vi "CG_Auswertung.vi"() -> ()   [LabVIEW 2020, in "Erweiterte Konfig.lvlib" / "CG-Check Konfig.lvlib"]
uses:
  CG-Check Konfig.lvlib
  CalEingaenge.ctl
  System Einstellungen V2/Aktioen FGV System Konstanten.ctl
  Aktion_CG-Check.ctl
  <vilib>/Utility/miscctls.llb/LVRowAndColumnTypeDef.ctl
  FT-IR/Span/Spanfaktor.lvlib
  Allgemein/allgemeine Sub-VIs.lvlib
  Sprachverwaltung/Sprachverwaltung.lvlib
  System Einstellungen V2/System Einstellungen V2.lvlib
panel:
  in  "Abbrechen":bool
  in  "Register":T1(tab)
  in  "Tabelle Span 1":string[][](table)
  in  "Tabelle Span 2":string[][](table)
  in  "Tabelle Span 3":string[][](table)
  in  "Tabelle Cal Gas O2":string[][](table)
  # "CG-Test Ergebnis"
  # "Komponente"
  # "Komponente"
  # "Komponente"
  # "Komponente"
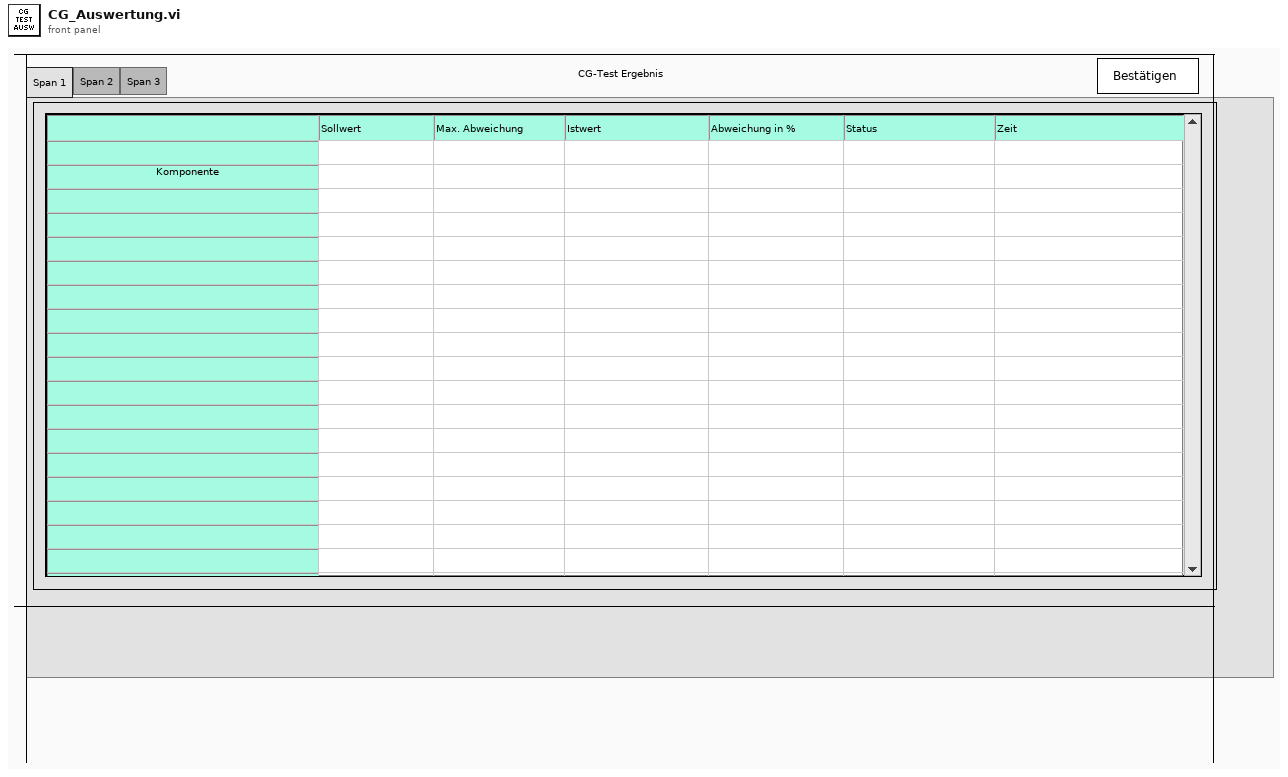
[diagram p1: front panel]
types:
  T1 = enum32{"Span 1", "Span 2", "Span 3", "Cal Gas O2"}
  T2 = typedef "System Einstellungen V2.lvlib/Aktioen FGV System Konstanten.ctl" = enum16{"lesen", "laden", "speichern", "Sprache"}
  T3 = typedef "Erweiterte Konfig.lvlib/CG-Check Konfig.lvlib/Aktion_CG-Check.ctl" = enum16{"lesen", "schreiben", "laden", "Komponente", "Aktive?", "speichern"}
  T4 = typedef "LVRowAndColumnTypeDef.ctl" = cluster{"Row":i32, "Column":i32}
  T5 = typedef "Erweiterte Konfig.lvlib/CG-Check Konfig.lvlib/CalEingaenge.ctl" = string[]
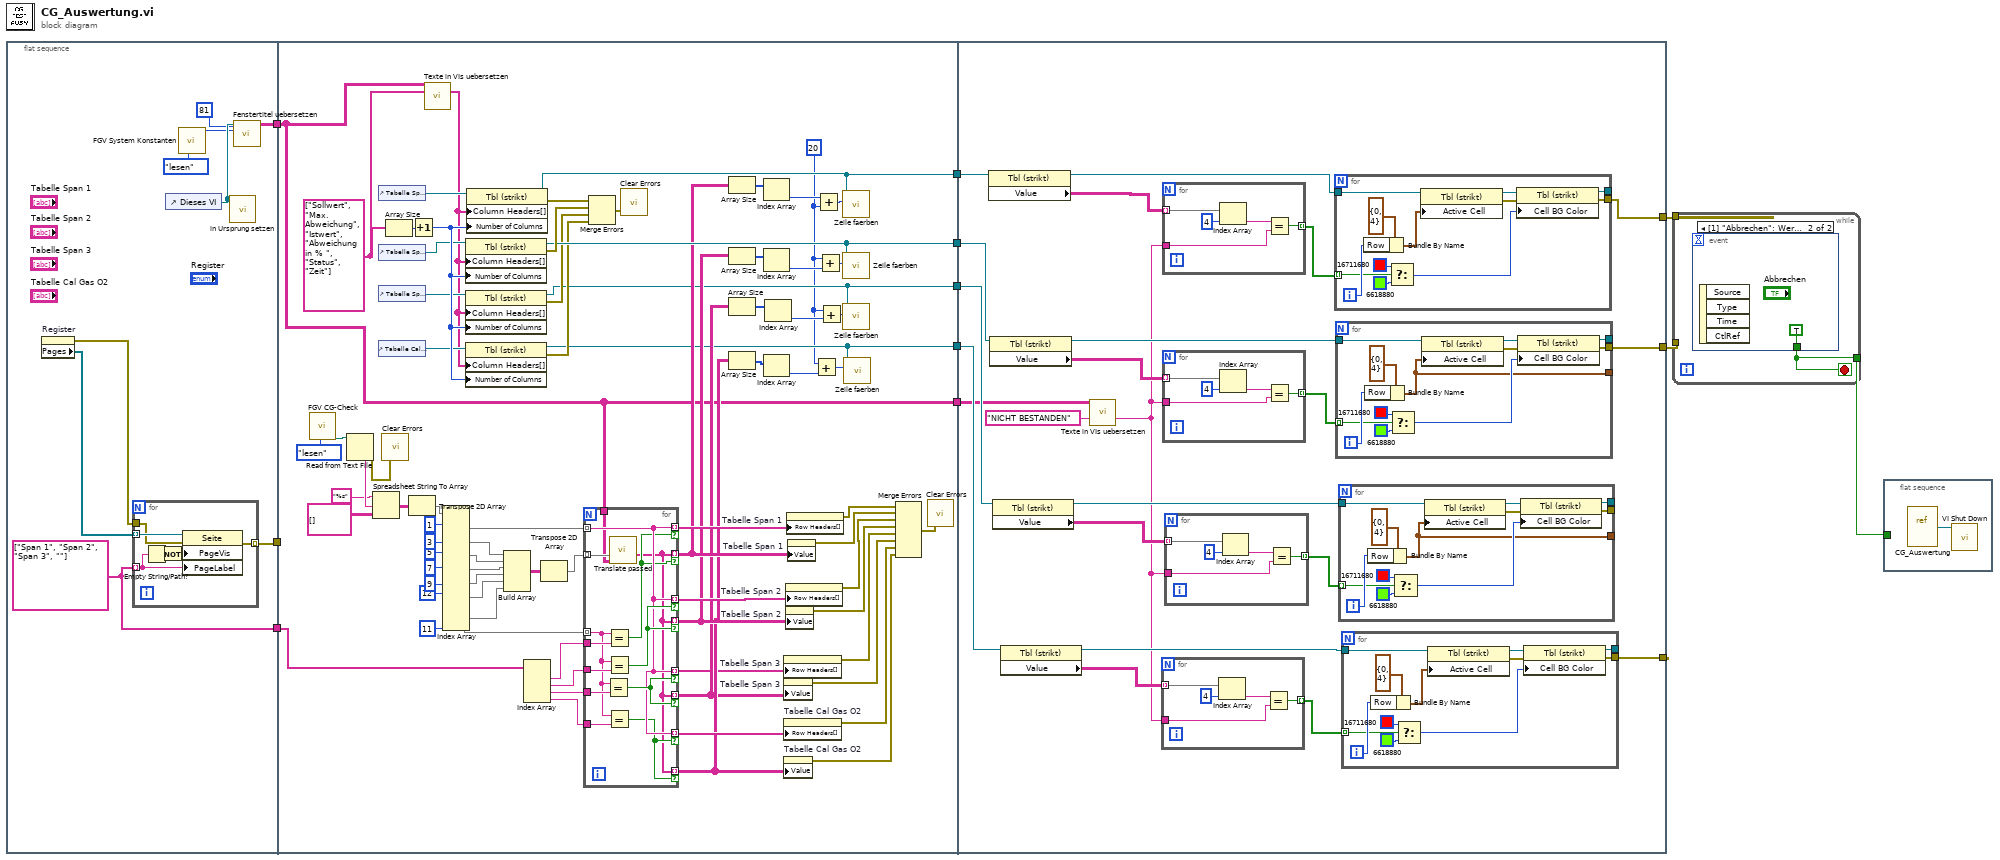
[diagram p0: block diagram]
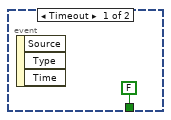
[diagram p2: hidden frame]
diagram:
  n1 = flat-sequence {
    tunnel: [w18] -> w5
    tunnel: [w17] -> w4
    tunnel: [w12] -> w2
    tunnel: [w66] -> w9
    tunnel: [w65] -> w8
    tunnel: [w35] -> w6
    tunnel: w5 -> [_]
    tunnel: w4 -> [w62]
    tunnel: [w34] -> w3
    tunnel: w2 -> [w27]
    tunnel: [w27] -> w1
    tunnel: [w131] -> w11
    tunnel: w9 -> [w139]
    tunnel: w8 -> [w138]
    tunnel: [w126] -> w7
    tunnel: w6 -> [w122]
    tunnel: [w127] -> _
    tunnel: w3 -> [w121]
    tunnel: w1 -> [w120]
    frame #0 {
      w17 = T5 ["Span 1", "Span 2", "Span 3", ""]
      n2 = property on="Register" class="RKElem (strikt)"() -> (error out=w20:errorcluster, "Pages"=w19:refnum<vi>[])  [unwired: 2 in, 1 out]
      n3 = for {
        tunnel: w19 -> [w26] mode=indexing
        tunnel: w20 -> [w25]
        tunnel: [w24] -> w18 mode=indexing
        tunnel: w17 -> [w23] mode=indexing
        n4 = Empty String/Path?(string/path=w23) -> (empty?=w22:bool)
        n5 = Not(x=w22) -> (.not. x?=w21:bool)
        n6 = property class="Seite"(reference=w26, error in=w25, "PageVis"=w21, "PageLabel"=w23) -> (error out=w24:errorcluster)  [unwired: 1 out]
      }
      n7 = control-ref of="Dieses VI"() -> (w16:refnum<vi>)
      n8 = call "FGV System Konstanten.vi"("Aktionen"=Aktioen_FGV_System_Konstanten."lesen") -> ("Sprachindex"=w13:u16)  [unwired: 6 in, 4 out]
      n9 = call "in Ursprung setzen.vi"("VI Referenz"=w16) -> ()  [unwired: 10 in, 1 out]
      n10 = call "Fenstertitel uebersetzen.vi"("Index (Seite)"=81, "Sprachauswahl"=w13, "Dieses VI"=w16) -> ("Sprachliste"=w12:string[][])  [unwired: 5 in, 3 out]
    }
    frame #1 {
      w29 = string[] ["Sollwert", "Max. Abweichung", "Istwert", "Abweichung in % ", "Status", "Zeit"] ("Spaltentitel[]")
      w32 = 20 ("y")
      n11 = call "FGV CG-Check.vi"("Aktion"=Aktion_CG-Check."lesen") -> ("Pfad:"=w78:path)  [unwired: 11 in, 7 out]
      n12 = Read from Text File(file (use dialog)=w78) -> (text=w104:string, error out=w77:errorcluster)  [unwired: 2 in, 3 out]
      n13 = Spreadsheet String To Array(format string="%s" ("Format-String"), spreadsheet string=w104, array type (2D Dbl)=string[][] []) -> (array=w101:string[][])  [unwired: 1 out]
      n14 = control-ref of="Tabelle Span 1"() -> (w40:refnum<vi>)
      n15 = control-ref of="Tabelle Span 2"() -> (w39:refnum<vi>)
      n16 = control-ref of="Tabelle Span 3"() -> (w38:refnum<vi>)
      n17 = control-ref of="Tabelle Cal Gas O2"() -> (w37:refnum<vi>)
      n18 = call <vilib>:"Clear Errors.vi"("error in (no error)"=w77) -> ()  [unwired: 5 in, 2 out]
      n19 = Array Size(array=w29) -> (size(s)=w75:i32)
      n20 = Transpose 2D Array(2D array=w101) -> (transposed array=w99:string[][])
      n21 = Increment(x=w75) -> (x+1=w47:i32)
      n22 = call "Texte in VIs uebersetzen.vi"("Sprachliste"=w27, "String-Array zum Übersetzen"=w29) -> ("String-Array zum Übersetzen"=w28:string[])  [unwired: 9 in, 4 out]
      n23 = Index Array(array=w99, index (row) #1=1 ("Index (Zeile)"), index (row) #2=3 ("Index (Zeile)"), index (row) #3=5 ("Index (Zeile)"), index (row) #4=7 ("Index (Zeile)"), index (row) #5=9 ("Index (Zeile)"), index (row) #6=12 ("Index (Zeile)"), index (row) #8=11 ("Index (Zeile)")) -> (element #1=w83:string[], element #2=w93:string[], element #3=w92:string[], element #4=w91:string[], element #5=w90:string[], element #6=w89:string[], element #7=w87:string[], element #8=w85:string[])  [unwired: 9 in]
      n24 = property on="Eigenschaftsknoten" class="Tbl (strikt)"(reference=w39, "Column Headers[]"=w28, "Number of Columns"=w47) -> (reference out=w65:refnum<vi>, error out=w73:errorcluster)  [unwired: 1 in]
      n25 = property on="Eigenschaftsknoten" class="Tbl (strikt)"(reference=w38, "Column Headers[]"=w28, "Number of Columns"=w47) -> (reference out=w35:refnum<vi>, error out=w64:errorcluster)  [unwired: 1 in]
      n26 = property on="Eigenschaftsknoten" class="Tbl (strikt)"(reference=w37, "Column Headers[]"=w28, "Number of Columns"=w47) -> (reference out=w34:refnum<vi>, error out=w46:errorcluster)  [unwired: 1 in]
      n27 = property on="Eigenschaftsknoten" class="Tbl (strikt)"(reference=w40, "Column Headers[]"=w28, "Number of Columns"=w47) -> (reference out=w66:refnum<vi>, error out=w74:errorcluster)  [unwired: 1 in]
      n28 = Build Array(w93, w92, w91, w90, w89, w87) -> (w88:string[][])
      n29 = Index Array(array=w62) -> (element #1=w61:string, element #2=w60:string, element #3=w59:string, element #4=w52:string)  [unwired: 4 in]
      n30 = Transpose 2D Array(2D array=w88) -> (transposed array=w84:string[][])
      n31 = for {
        tunnel: w61 -> [w117]
        tunnel: w85 -> [w112] mode=indexing
        tunnel: w84 -> [w107] mode=indexing
        tunnel: w83 -> [w110] mode=indexing
        tunnel: [w106] -> w44 mode=indexing if=w114
        tunnel: [w110] -> w57 mode=indexing if=w114
        tunnel: [w110] -> w80 mode=indexing if=w108
        tunnel: [w106] -> w45 mode=indexing if=w108
        tunnel: w60 -> [w116]
        tunnel: [w110] -> w30 mode=indexing if=w113
        tunnel: [w106] -> w42 mode=indexing if=w113
        tunnel: w59 -> [w115]
        tunnel: w52 -> [w111]
        tunnel: [w106] -> w43 mode=indexing if=w109
        tunnel: [w110] -> w49 mode=indexing if=w109
        tunnel: w27 -> [w105]
        n32 = Equal?(x=w112, y=w115) -> (x = y?=w113:bool)
        n33 = Equal?(x=w112, y=w117) -> (x = y?=w108:bool)
        n34 = Equal?(x=w112, y=w116) -> (x = y?=w114:bool)
        n35 = Equal?(x=w112, y=w111) -> (x = y?=w109:bool)
        n36 = call "Translate passed.vi"("Sprachliste"=w105, "Array (Eingang)"=w107) -> ("Array (Ausgang)"=w106:string[])  [unwired: 9 in]
      }
      n37 = Merge Errors(w74, w73, w64, w46) -> (w72:errorcluster)
      n38 = call <vilib>:"Clear Errors.vi"("error in (no error)"=w72) -> ()  [unwired: 5 in, 2 out]
      n39 = Array Size(array=w45) -> (size(s)=w69:i32[])
      n40 = Array Size(array=w44) -> (size(s)=w71:i32[])
      n41 = Array Size(array=w42) -> (size(s)=w41:i32[])
      n42 = Array Size(array=w43) -> (size(s)=w48:i32[])
      n43 = Index Array(array=w69) -> (element=w67:i32)  [unwired: 1 in]
      n44 = Index Array(array=w71) -> (element=w70:i32)  [unwired: 1 in]
      n45 = Index Array(array=w48) -> (element=w33:i32)  [unwired: 1 in]
      n46 = Index Array(array=w41) -> (element=w36:i32)  [unwired: 1 in]
      n47 = property on="Tabelle Span 3" class="Tbl (strikt)"("Row Headers[]"=w30) -> (error out=w54:errorcluster)  [unwired: 2 in, 1 out]
      n48 = property on="Tabelle Span 3" class="Tbl (strikt)"("Value"=w42) -> (error out=w53:errorcluster)  [unwired: 2 in, 1 out]
      n49 = property on="Tabelle Cal Gas O2" class="Tbl (strikt)"("Row Headers[]"=w49) -> (error out=w51:errorcluster)  [unwired: 2 in, 1 out]
      n50 = property on="Tabelle Cal Gas O2" class="Tbl (strikt)"("Value"=w43) -> (error out=w50:errorcluster)  [unwired: 2 in, 1 out]
      n51 = property on="Tabelle Span 2" class="Tbl (strikt)"("Row Headers[]"=w57) -> (error out=w56:errorcluster)  [unwired: 2 in, 1 out]
      n52 = property on="Tabelle Span 2" class="Tbl (strikt)"("Value"=w44) -> (error out=w55:errorcluster)  [unwired: 2 in, 1 out]
      n53 = property on="Tabelle Span 1" class="Tbl (strikt)"("Row Headers[]"=w80) -> (error out=w81:errorcluster)  [unwired: 2 in, 1 out]
      n54 = property on="Tabelle Span 1" class="Tbl (strikt)"("Value"=w45) -> (error out=w82:errorcluster)  [unwired: 2 in, 1 out]
      n55 = Add(x=w32, y=w33) -> (x+y=w31:i32)
      n56 = Add(x=w67, y=w32) -> (x+y=w68:i32)
      n57 = Add(x=w32, y=w70) -> (x+y=w76:i32)
      n58 = Add(x=w32, y=w36) -> (x+y=w63:i32)
      n59 = call "Zeile faerben.vi"("Anzahl"=w68, "Table (Eingang)"=w66) -> ()  [unwired: 9 in, 1 out]
      n60 = call "Zeile faerben.vi"("Anzahl"=w76, "Table (Eingang)"=w65) -> ()  [unwired: 9 in, 1 out]
      n61 = call "Zeile faerben.vi"("Anzahl"=w63, "Table (Eingang)"=w35) -> ()  [unwired: 9 in, 1 out]
      n62 = call "Zeile faerben.vi"("Anzahl"=w31, "Table (Eingang)"=w34) -> ()  [unwired: 9 in, 1 out]
      n63 = Merge Errors(w81, w82, w56, w55, w54, w53, w51, w50) -> (w58:errorcluster)
      n64 = call <vilib>:"Clear Errors.vi"("error in (no error)"=w58) -> ()  [unwired: 5 in, 2 out]
    }
    frame #2 {
      n65 = property class="Tbl (strikt)"(reference=w139) -> (reference out=w136:refnum<vi>, "Value"=w137:string[][])  [unwired: 1 in, 1 out]
      n66 = property class="Tbl (strikt)"(reference=w138) -> (reference out=w132:refnum<vi>, "Value"=w134:string[][])  [unwired: 1 in, 1 out]
      n67 = property class="Tbl (strikt)"(reference=w122) -> (reference out=w125:refnum<vi>, "Value"=w123:string[][])  [unwired: 1 in, 1 out]
      n68 = property class="Tbl (strikt)"(reference=w121) -> (reference out=w128:refnum<vi>, "Value"=w129:string[][])  [unwired: 1 in, 1 out]
      n69 = call "Texte in VIs uebersetzen.vi"("Sprachliste"=w120, "String zum Übersetzen"="NICHT BESTANDEN" ("y")) -> ("String zum Übersetzen"=w118:string)  [unwired: 9 in, 4 out]
      n70 = for {
        tunnel: w129 -> [w173] mode=indexing
        tunnel: [w170] -> w130 mode=indexing
        tunnel: w118 -> [w169]
        n71 = Index Array(array=w173, index=4 ("Index")) -> (element=w171:string)
        n72 = Equal?(x=w171, y=w169) -> (x = y?=w170:bool)
      }
      n73 = for {
        tunnel: w137 -> [w207] mode=indexing
        tunnel: [w204] -> w135 mode=indexing
        tunnel: w118 -> [w203]
        n74 = Index Array(array=w207, index=4 ("Index")) -> (element=w205:string)
        n75 = Equal?(x=w205, y=w203) -> (x = y?=w204:bool)
      }
      n76 = for {
        tunnel: w134 -> [w190] mode=indexing
        tunnel: [w187] -> w133 mode=indexing
        tunnel: w118 -> [w186]
        n77 = Index Array(array=w190, index=4 ("Index")) -> (element=w188:string)
        n78 = Equal?(x=w188, y=w186) -> (x = y?=w187:bool)
      }
      n79 = for {
        tunnel: w123 -> [w156] mode=indexing
        tunnel: [w153] -> w124 mode=indexing
        tunnel: w118 -> [w152]
        n80 = Index Array(array=w156, index=4 ("Index")) -> (element=w154:string)
        n81 = Equal?(x=w154, y=w152) -> (x = y?=w153:bool)
      }
      n82 = for {
        tunnel: w136 -> [w202]
        tunnel: w135 -> [w196] mode=indexing
        tunnel: [w195] -> _
        tunnel: [w194] -> w131
        i -> [w197]
        n83 = Bundle By Name(cluster=T4 {"Row"=0, "Column"=4} ("Aktive Zelle:Aktive Zelle"), "Row"=w197) -> (w191:T4)
        n84 = Select(t=u32 16711680, s=w196, f=u32 6618880) -> (s? t:f=w198:u32)
        n85 = property class="Tbl (strikt)"(reference=w202, "Active Cell"=w191) -> (reference out=w200:refnum<vi>, error out=w199:errorcluster)  [unwired: 1 in]
        n86 = property class="Tbl (strikt)"(reference=w200, error in=w199, "Cell BG Color"=w198) -> (reference out=w195:refnum<vi>, error out=w194:errorcluster)
      }
      n87 = for {
        tunnel: w132 -> [w185]
        tunnel: w133 -> [w179] mode=indexing
        tunnel: [w178] -> _
        tunnel: [w177] -> w126
        tunnel: [w174] -> _
        i -> [w180]
        n88 = Bundle By Name(cluster=T4 {"Row"=0, "Column"=4} ("Aktive Zelle:Aktive Zelle"), "Row"=w180) -> (w174:T4)
        n89 = Select(t=u32 16711680, s=w179, f=u32 6618880) -> (s? t:f=w181:u32)
        n90 = property class="Tbl (strikt)"(reference=w185, "Active Cell"=w174) -> (reference out=w183:refnum<vi>, error out=w182:errorcluster)  [unwired: 1 in]
        n91 = property class="Tbl (strikt)"(reference=w183, error in=w182, "Cell BG Color"=w181) -> (reference out=w178:refnum<vi>, error out=w177:errorcluster)
      }
      n92 = for {
        tunnel: w125 -> [w151]
        tunnel: w124 -> [w145] mode=indexing
        tunnel: [w144] -> _
        tunnel: [w143] -> _
        tunnel: [w140] -> _
        i -> [w146]
        n93 = Bundle By Name(cluster=T4 {"Row"=0, "Column"=4} ("Aktive Zelle:Aktive Zelle"), "Row"=w146) -> (w140:T4)
        n94 = Select(t=u32 16711680, s=w145, f=u32 6618880) -> (s? t:f=w147:u32)
        n95 = property class="Tbl (strikt)"(reference=w151, "Active Cell"=w140) -> (reference out=w149:refnum<vi>, error out=w148:errorcluster)  [unwired: 1 in]
        n96 = property class="Tbl (strikt)"(reference=w149, error in=w148, "Cell BG Color"=w147) -> (reference out=w144:refnum<vi>, error out=w143:errorcluster)
      }
      n97 = for {
        tunnel: w128 -> [w168]
        tunnel: w130 -> [w162] mode=indexing
        tunnel: [w161] -> _
        tunnel: [w160] -> w127
        i -> [w163]
        n98 = Bundle By Name(cluster=T4 {"Row"=0, "Column"=4} ("Aktive Zelle:Aktive Zelle"), "Row"=w163) -> (w157:T4)
        n99 = Select(t=u32 16711680, s=w162, f=u32 6618880) -> (s? t:f=w164:u32)
        n100 = property class="Tbl (strikt)"(reference=w168, "Active Cell"=w157) -> (reference out=w166:refnum<vi>, error out=w165:errorcluster)  [unwired: 1 in]
        n101 = property class="Tbl (strikt)"(reference=w166, error in=w165, "Cell BG Color"=w164) -> (reference out=w161:refnum<vi>, error out=w160:errorcluster)
      }
    }
  }
  n102 = while {
    tunnel: w11 -> [_]
    tunnel: [w208] -> w10
    tunnel: w7 -> [_]
    stop <- w208 stop-if-true
    n103 = event shown="[1] \"Abbrechen\": Wertänderung" {
      selector: _ -> [_ _]
      dyn-events: _ -> [_ _]
      timeout: _ -> [_ _]
      tunnel: [FALSE ("Abbrechen") TRUE ("Abbrechen")] -> w208
      event Timeout {
        n104 = event-data() -> ()  [unwired: 1 in, 3 out]
      }
      event "Abbrechen": Value Change {
        n105 = event-data() -> ()  [unwired: 1 in, 4 out]
      }
    }
  }
  n106 = flat-sequence {
    tunnel: w10 -> [_]
    frame #0 {
      n107 = vi-ref "CG_Auswertung.vi"() -> (w211:refnum<vi>)
      n108 = call "VI Shut Down.vi"("VI Referenz"=w211) -> ()  [unwired: 11 in]
    }
  }
